vi "New Setup - RF Patch Prompt.vi"(9 "Motion":bool, 10 "NewSetup":T1) -> (2 "Dialog Prompt":string)   [LabVIEW 2018]
uses:
  PatchNewTestStep.ctl
  RF Direction.ctl
  PolarizationSelect.ctl
  APARMainSubvis/VXM Public API/singleAxisMoveDef.ctl
  APARMainSubvis/VXM Public API/mmWaveAxis.ctl
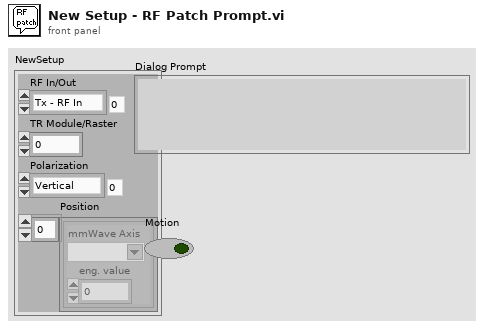
[diagram p1: front panel]
types:
  T1 = typedef "PatchNewTestStep.ctl" = cluster{"RF In/Out":T2, "TR Module/Raster":i32, "Polarization":T3, "Position":T4[]}
  T2 = typedef "RF Direction.ctl" = enum16{"Tx - RF In", "Rx - RF Out"}
  T3 = typedef "PolarizationSelect.ctl" = enum16{"Vertical", "Horizontal"}
  T4 = typedef "singleAxisMoveDef.ctl" = cluster{"mmWave Axis":T5, "eng. value":dbl}
  T5 = typedef "mmWaveAxis.ctl" = string
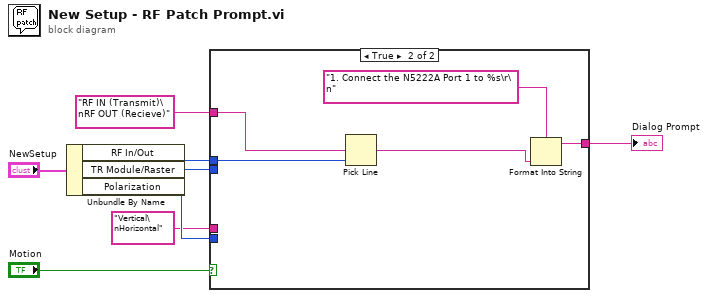
[diagram p0: block diagram]
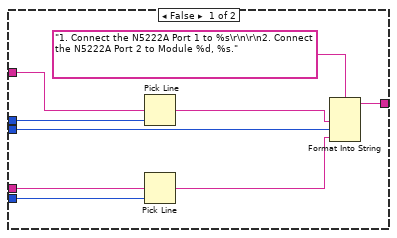
[diagram p2: hidden frame]
diagram:
  n1 = Unbundle By Name("NewSetup") -> ("RF In/Out"=w7:T2, "TR Module/Raster"=w5:i32, "Polarization"=w4:T3)
  n2 = case shown="True" "Motion" {
    tunnel: w7 -> [w17 w22]
    tunnel: "RF IN (Transmit)\nRF OUT (Recieve)" ("multi-line string") -> [w16 w21]
    tunnel: w5 -> [w13 _]
    tunnel: w4 -> [w12 _]
    tunnel: "Vertical\nHorizontal" ("multi-line string") -> [w11 _]
    tunnel: [w9 w18] -> w2
    frame False {
      n3 = Pick Line(multi-line string=w16, line index=w17) -> (output string=w14:string)  [unwired: 1 in]
      n4 = Pick Line(multi-line string=w11, line index=w12) -> (output string=w10:string)  [unwired: 1 in]
      n5 = Format Into String(format string="1. Connect the N5222A Port 1 to %s\r\n\r\n2. Connect the N5222A Port 2 to Module %d, %s.", w14, w13, w10) -> (resulting string=w9:string)  [unwired: 2 in, 1 out]
    }
    frame True {
      n6 = Pick Line(multi-line string=w21, line index=w22) -> (output string=w19:string)  [unwired: 1 in]
      n7 = Format Into String(format string="1. Connect the N5222A Port 1 to %s\r\n", w19) -> (resulting string=w18:string)  [unwired: 2 in, 1 out]
    }
  }
  "Dialog Prompt" <- w2
